vi "Main.vi"(8 "error in (no error)":errorcluster, 11 "RSABase in":refnum<class "RSA.lvclass">) -> (0 "error out":errorcluster, 3 "component":refnum<class "RSA.lvclass">)   [LabVIEW 2012, in "RSA.lvclass"]
doc: "Main VI of the component."
uses:
  RSA.lvclass
  <vilib>/Distrio/Murmex/Murmex/command_enum.ctl
  starting shape.ctl
  RSA.lvclass/RSA.ctl
  <vilib>/Distrio/Murmex/InitialiseMessage/InitialiseMessage.lvclass
  <vilib>/Distrio/Murmex/TerminateMessage/TerminateMessage.lvclass
  <vilib>/Distrio/Murmex/ConfigureMessage/ConfigureMessage.lvclass
  <vilib>/Distrio/Murmex/StartMessage/StartMessage.lvclass
  <vilib>/Distrio/Murmex/Murmex/update_cluster.ctl
  <vilib>/Distrio/Murmex/ResetMessage/ResetMessage.lvclass
  <vilib>/Distrio/Murmex/Murmex/Set configure at initialise.vi
  <vilib>/Distrio/Murmex/Murmex/Set log reference.vi
  <vilib>/Distrio/Murmex/Murmex/Set VI reference.vi
  <vilib>/Distrio/Murmex/Murmex/Get ID.vi
  <vilib>/Distrio/Murmex/Murmex/Murmex.lvclass
  <vilib>/Distrio/Murmex/Message/Message.lvclass
panel:
  in  "button::stop":bool
  in  "button::reset":bool
  in  "button::start":bool
  in  "button::quit":bool
  in  "Tab Control":enum32{"Settings", "Indicators", "Debug"}(tab)
  in  "Starting shape":T1=enum."Midrange"
  in  "BC buffer size":i32=12
  in  "Wait time":dbl[unit]=50.0
  in  "stop after":i32=500
  in  "Iterations until BC":i32=5000
  in  "Search Range [%]":dbl(knob)=100.0 min=0.0 max=100.0 step=5.0 scale=0.0..100.0
  in  "Optimisation name":string="bob"
  out "current MF":cluster{"Y":dbl[], "Y":dbl[]}[](graph)
  out "unsuccessfull iterations":i32
  out "successfull iterations":i32
  out "current Merit Factor":dbl
  out "Iterations since last improvement":i32
  out "max Merit Factor":dbl
  out "BC on":bool
  out "MF standard deviation":dbl
  out "best MF":cluster{"Y":dbl[], "Y":dbl[]}[](graph)
  out "BC counter":i32
  out "log":string="\r\n11:11:41.970 05/12/2013: initialise from AOTF to AOTF\r\n11:11:42.586 05/12/2013: inform from AOTF to AOTF\r\n11:11:43.913 05/12/2013: update from AOTF to AOTF\r\n11:11:45.142 05/12/2013: generic (shutter_off) from AOTF to AOTF\r\n11:11:45.270 05/12/2013: generic (shutter_on) from AOTF to AOTF\r\n11:11:45.902 05/12/2013: generic (shutter_off) from AOTF to AOTF\r\n11:11:45.932 05/12/2013: inspect from AOTF to AOTF\r\n11:11:48.013 05/12/2013: configure from AOTF to AOTF\r\n11:11:52.003 05/12/2013: inform from AOTF to AOTF\r\n11:11:58.521 05/12/2013: initialise from AOTF to AOTF\r\n11:11:58.561 05/12/2013: inform from AOTF to AOTF\r\n11:11:58.695 05/12/2013: inform from AOTF to AOTF\r\n11:12:02.089 05/12/2013: update from AOTF to AOTF\r\n11:12:02.308 05/12/2013: inspect from AOTF to AOTF\r\n11:12:02.364 05/12/2013: inform from AOTF to AOTF\r\n11:12:05.062 05/12/2013: generic (shutter_on) from AOTF to AOTF\r\n11:12:06.690 05/12/2013: update from AOTF to AOTF\r\n11:12:06.909 05/12/2013: inspect from AOTF to AOTF\r\n11:12:06.964 05/12/2013: inform from AOTF to AOTF\r\n11:12:07.770 05/12/2013: update from AOTF to AOTF\r\n11:12:07.989 05/12/2013: inspect from AOTF to AOTF\r\n11:12:08.044 05/12/2013: inform from AOTF to AOTF\r\n11:12:08.627 05/12/2013: update from AOTF to AOTF\r\n11:12:08.846 05/12/2013: inspect from AOTF to AOTF\r\n11:12:08.900 05/12/2013: inform from AOTF to AOTF\r\n11:12:09.290 05/12/2013: update from AOTF to AOTF\r\n11:12:09.508 05/12/2013: inspect from AOTF to AOTF\r\n11:12:09.563 05/12/2013: inform from AOTF to AOTF\r\n11:12:10.154 05/12/2013: update from AOTF to AOTF\r\n11:12:10.373 05/12/2013: inspect from AOTF to AOTF\r\n11:12:10.430 05/12/2013: inform from AOTF to AOTF\r\n11:12:20.953 05/12/2013: update from AOTF to AOTF\r\n11:12:21.172 05/12/2013: inspect from AOTF to AOTF\r\n11:12:21.227 05/12/2013: inform from AOTF to AOTF\r\n11:12:22.057 05/12/2013: update from AOTF to AOTF\r\n11:12:22.276 05/12/2013: inspect from AOTF to AOTF\r\n11:12:22.330 05/12/2013: inform from AOTF to AOTF\r\n11:12:22.841 05/12/2013: update from AOTF to AOTF\r\n11:12:23.060 05/12/2013: inspect from AOTF to AOTF\r\n11:12:23.114 05/12/2013: inform from AOTF to AOTF\r\n11:12:23.449 05/12/2013: update from AOTF to AOTF\r\n11:12:23.668 05/12/2013: inspect from AOTF to AOTF\r\n11:12:23.724 05/12/2013: inform from AOTF to AOTF\r\n11:12:24.514 05/12/2013: update from AOTF to AOTF\r\n11:12:24.733 05/12/2013: inspect from AOTF to AOTF\r\n11:12:24.789 05/12/2013: inform from AOTF to AOTF\r\n11:12:25.098 05/12/2013: update from AOTF to AOTF\r\n11:12:25.317 05/12/2013: inspect from AOTF to AOTF\r\n11:12:25.371 05/12/2013: inform from AOTF to AOTF\r\n11:12:26.482 05/12/2013: update from AOTF to AOTF\r\n11:12:26.701 05/12/2013: inspect from AOTF to AOTF\r\n11:12:26.755 05/12/2013: inform from AOTF to AOTF\r\n11:12:27.154 05/12/2013: update from AOTF to AOTF\r\n11:12:27.373 05/12/2013: inspect from AOTF to AOTF\r\n11:12:27.428 05/12/2013: inform from AOTF to AOTF\r\n11:12:27.666 05/12/2013: update from AOTF to AOTF\r\n11:12:27.885 05/12/2013: inspect from AOTF to AOTF\r\n11:12:27.944 05/12/2013: inform from AOTF to AOTF\r\n11:12:33.380 05/12/2013: update from AOTF to AOTF\r\n11:12:33.484 05/12/2013: update from AOTF to AOTF\r\n11:12:33.603 05/12/2013: inspect from AOTF to AOTF\r\n11:12:33.611 05/12/2013: update from AOTF to AOTF\r\n11:12:33.684 05/12/2013: update from AOTF to AOTF\r\n11:12:33.740 05/12/2013: update from AOTF to AOTF\r\n11:12:33.827 05/12/2013: inspect from AOTF to AOTF\r\n11:12:33.835 05/12/2013: update from AOTF to AOTF\r\n11:12:33.897 05/12/2013: inform from AOTF to AOTF\r\n11:12:33.903 05/12/2013: update from AOTF to AOTF\r\n11:12:33.940 05/12/2013: update from AOTF to AOTF\r\n11:12:34.085 05/12/2013: update from AOTF to AOTF\r\n11:12:34.119 05/12/2013: inspect from AOTF to AOTF\r\n11:12:34.292 05/12/2013: update from AOTF to AOTF\r\n11:12:34.336 05/12/2013: inspect from AOTF to AOTF\r\n11:12:34.553 05/12/2013: inspect from AOTF to AOTF\r\n11:12:34.608 05/12/2013: inform from AOTF to AOTF\r\n11:12:34.739 05/12/2013: update from AOTF to AOTF\r\n11:12:34.771 05/12/2013: update from AOTF to AOTF\r\n11:12:34.826 05/12/2013: inspect from AOTF to AOTF\r\n11:12:34.834 05/12/2013: update from AOTF to AOTF\r\n11:12:34.867 05/12/2013: update from AOTF to AOTF\r\n11:12:34.931 05/12/2013: update from AOTF to AOTF\r\n11:12:34.979 05/12/2013: update from AOTF to AOTF\r\n11:12:35.003 05/12/2013: update from AOTF to AOTF\r\n11:12:35.027 05/12/2013: update from AOTF to AOTF\r\n11:12:35.041 05/12/2013: update from AOTF to AOTF\r\n11:12:35.051 05/12/2013: inspect from AOTF to AOTF\r\n11:12:35.066 05/12/2013: update from AOTF to AOTF\r\n11:12:35.116 05/12/2013: update from AOTF to AOTF\r\n11:12:35.171 05/12/2013: update from AOTF to AOTF\r\n11:12:35.211 05/12/2013: update from AOTF to AOTF\r\n11:12:35.273 05/12/2013: inspect from AOTF to AOTF\r\n11:12:35.287 05/12/2013: update from AOTF to AOTF\r\n11:12:35.475 05/12/2013: update from AOTF to AOTF\r\n11:12:35.495 05/12/2013: inspect from AOTF to AOTF\r\n11:12:35.549 05/12/2013: inform from AOTF to AOTF\r\n11:12:35.764 05/12/2013: inspect from AOTF to AOTF\r\n11:12:35.819 05/12/2013: inform from AOTF to AOTF\r\n11:12:35.861 05/12/2013: update from AOTF to AOTF\r\n11:12:35.877 05/12/2013: inform from AOTF to AOTF\r\n11:12:35.947 05/12/2013: update from AOTF to AOTF\r\n11:12:36.067 05/12/2013: update from AOTF to AOTF\r\n11:12:36.100 05/12/2013: inspect from AOTF to AOTF\r\n11:12:36.235 05/12/2013: update from AOTF to AOTF\r\n11:12:36.317 05/12/2013: inspect from AOTF to AOTF\r\n11:12:36.371 05/12/2013: inform from AOTF to AOTF\r\n11:12:36.587 05/12/2013: inspect from AOTF to AOTF\r\n11:12:36.771 05/12/2013: update from AOTF to AOTF\r\n11:12:36.804 05/12/2013: inspect from AOTF to AOTF\r\n11:12:37.020 05/12/2013: inspect from AOTF to AOTF\r\n11:12:37.238 05/12/2013: inspect from AOTF to AOTF\r\n11:12:37.456 05/12/2013: inspect from AOTF to AOTF\r\n11:12:37.673 05/12/2013: inspect from AOTF to AOTF\r\n11:12:37.891 05/12/2013: inspect from AOTF to AOTF\r\n11:12:37.946 05/12/2013: inform from AOTF to AOTF\r\n11:12:38.161 05/12/2013: inspect from AOTF to AOTF\r\n11:12:38.379 05/12/2013: inspect from AOTF to AOTF\r\n11:12:38.597 05/12/2013: inspect from AOTF to AOTF\r\n11:12:38.815 05/12/2013: inspect from AOTF to AOTF\r\n11:12:38.871 05/12/2013: inform from AOTF to AOTF\r\n11:12:39.086 05/12/2013: inspect from AOTF to AOTF\r\n11:12:39.303 05/12/2013: inspect from AOTF to AOTF\r\n11:12:39.363 05/12/2013: inform from AOTF to AOTF\r\n11:12:39.417 05/12/2013: inform from AOTF to AOTF\r\n11:12:39.633 05/12/2013: inspect from AOTF to AOTF\r\n11:12:39.852 05/12/2013: inspect from AOTF to AOTF\r\n11:12:40.069 05/12/2013: inspect from AOTF to AOTF\r\n11:12:40.124 05/12/2013: inform from AOTF to AOTF\r\n11:12:40.339 05/12/2013: inspect from AOTF to AOTF\r\n11:12:40.395 05/12/2013: inform from AOTF to AOTF\r\n11:12:40.448 05/12/2013: inform from AOTF to AOTF\r\n11:12:40.663 05/12/2013: inspect from AOTF to AOTF\r\n11:12:40.718 05/12/2013: inform from AOTF to AOTF\r\n11:12:40.770 05/12/2013: inform from AOTF to AOTF\r\n11:12:40.824 05/12/2013: inform from AOTF to AOTF\r\n11:12:40.877 05/12/2013: inform from AOTF to AOTF\r\n11:12:40.930 05/12/2013: inform from AOTF to AOTF\r\n11:12:40.982 05/12/2013: inform from AOTF to AOTF\r\n11:12:41.034 05/12/2013: inform from AOTF to AOTF\r\n11:12:41.092 05/12/2013: inform from AOTF to AOTF\r\n11:12:41.144 05/12/2013: inform from AOTF to AOTF\r\n11:12:41.196 05/12/2013: inform from AOTF to AOTF\r\n11:12:41.249 05/12/2013: inform from AOTF to AOTF\r\n11:12:41.307 05/12/2013: inform from AOTF to AOTF\r\n11:12:41.366 05/12/2013: inform from AOTF to AOTF\r\n11:12:41.424 05/12/2013: inform from AOTF to AOTF\r\n11:12:41.478 05/12/2013: inform from AOTF to AOTF\r\n11:12:41.533 05/12/2013: inform from AOTF to AOTF\r\n11:12:41.589 05/12/2013: inform from AOTF to AOTF\r\n11:12:42.246 05/12/2013: terminate from AOTF to AOTF"
  in  "ID":string="RSA"
  in  "command":T2
  in  "Generic command":string
  in  "button::configure":bool
  in  "button::send":bool
  out "terminate?":bool=TRUE
  # "RSA settings"
  # "Save settings"
  # "Bleaching compensation"
  # "Iterations"
  # "Merit Factor"
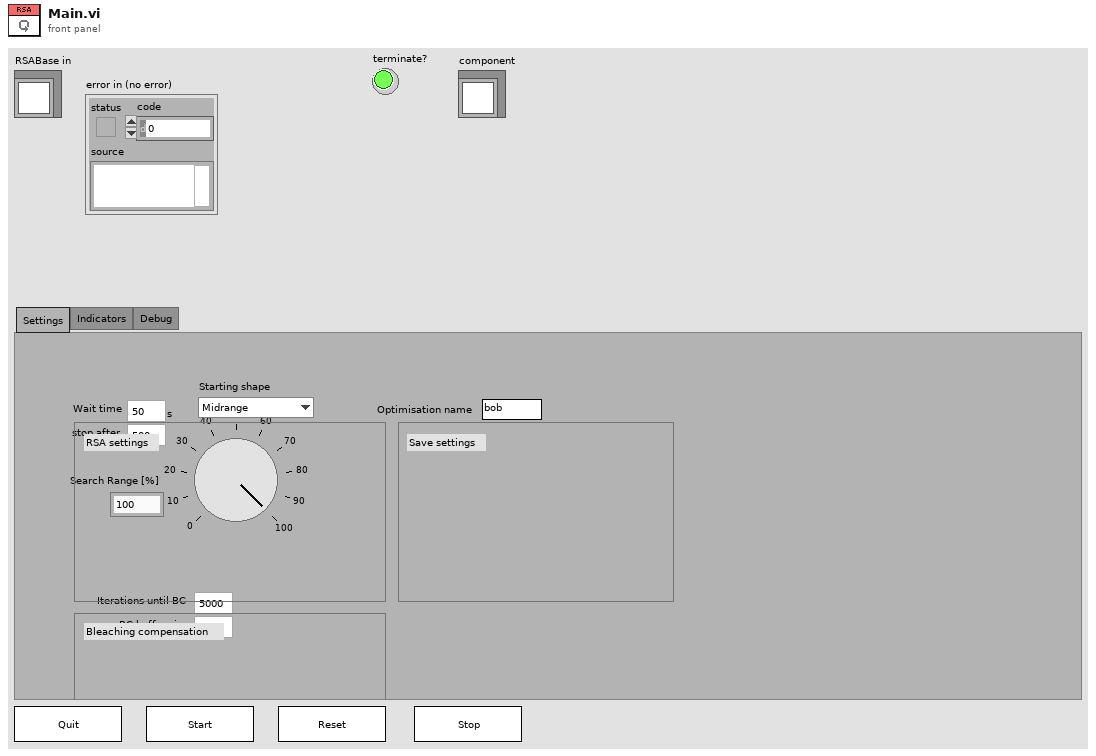
[diagram p1: front panel]
types:
  T1 = typedef "RSA.lvclass/starting shape.ctl" = enum16{"Load shape", "Midrange"}
  T2 = typedef "Murmex.lvlib/Murmex.lvclass/command_enum.ctl" = enum16{"null", "initialise", "reset", "terminate", "acknowledge", "update", "inspect", "inform", "proceed", "start", "stop", "fetch", "configure", "generic"}
  T3 = typedef "Murmex.lvlib/Murmex.lvclass/update_cluster.ctl" = cluster{"target ID":string, "key chains":string[], "values":variant[]}
  T4 = enum8{"Enabled", "Disabled", "Disabled and Grayed Out"}
  T5 = typedef "Murmex.lvclass/command_enum.ctl" = enum16{"null", "initialise", "reset", "terminate", "acknowledge", "update", "inspect", "inform", "proceed", "start", "stop", "fetch", "configure", "generic"}
  T6 = typedef "Murmex.lvclass/Event type enumerations.ctl" = enum16{"before", "after"}
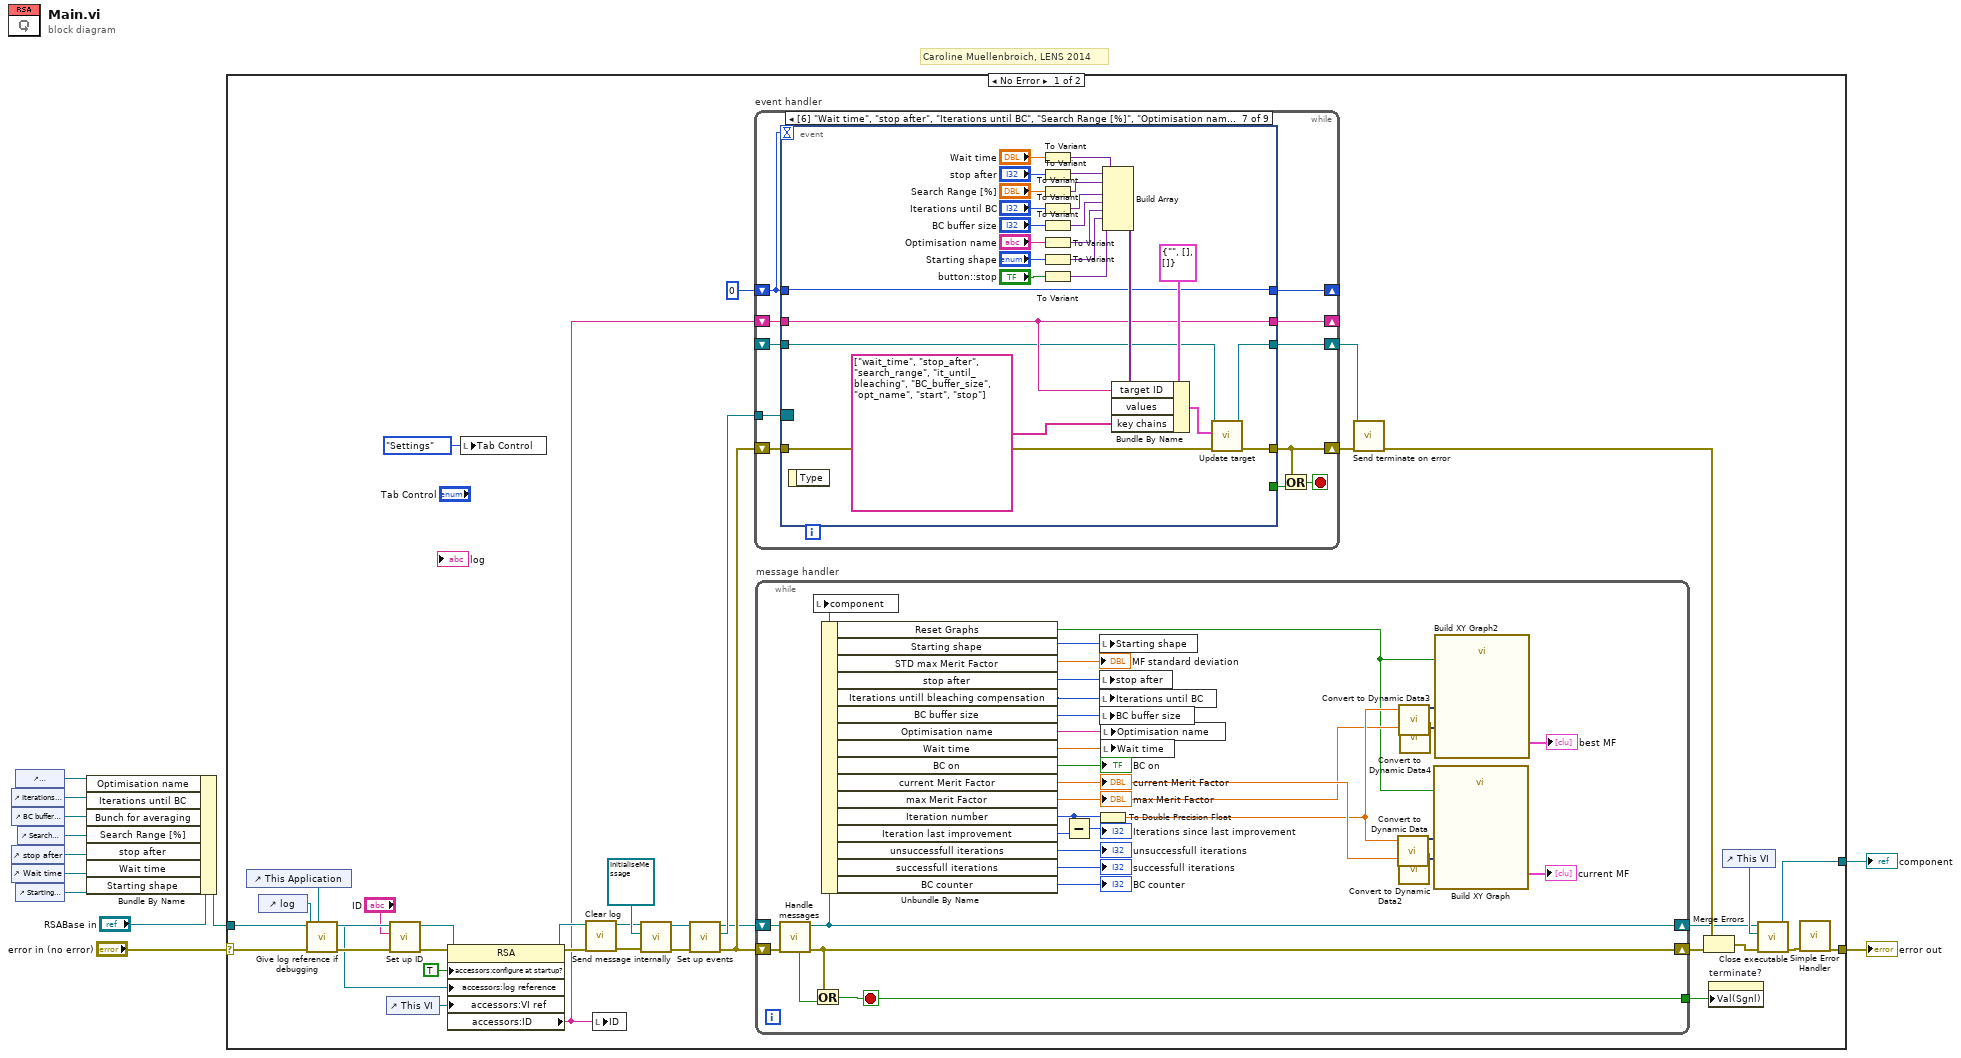
[diagram p0: block diagram]
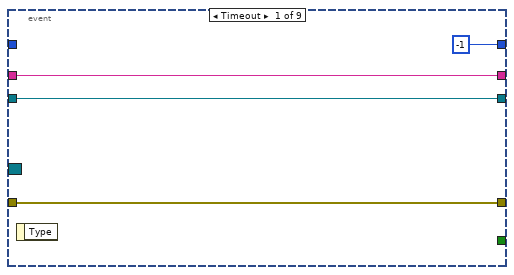
[diagram p2: hidden frame]
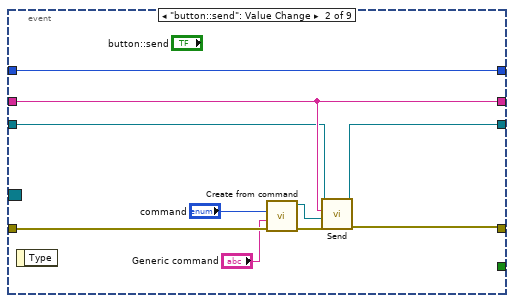
[diagram p3: hidden frame]
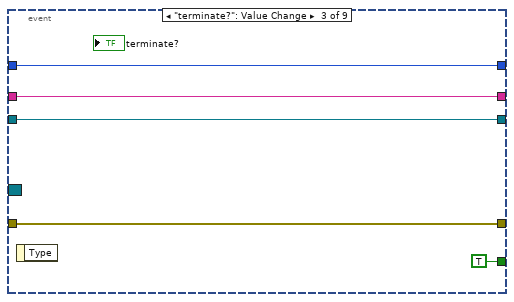
[diagram p4: hidden frame]
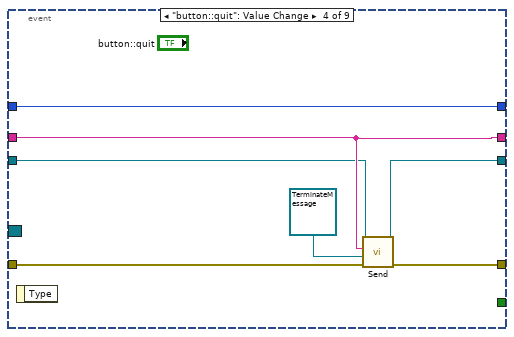
[diagram p5: hidden frame]
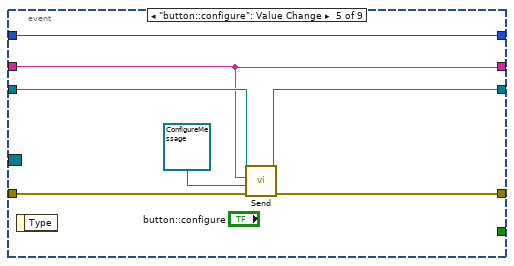
[diagram p6: hidden frame]
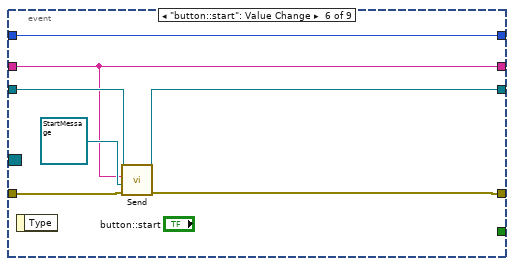
[diagram p7: hidden frame]
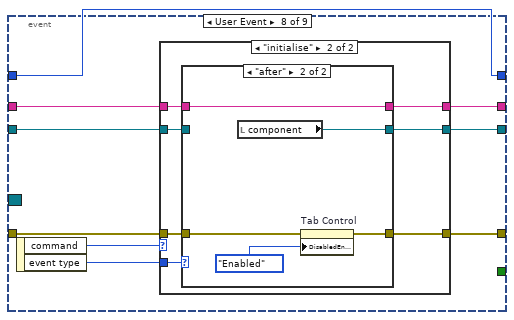
[diagram p8: hidden frame]
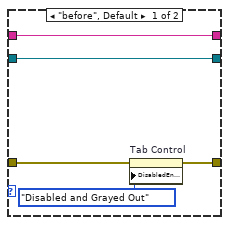
[diagram p10: hidden frame]
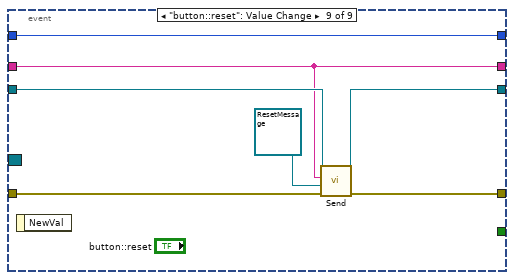
[diagram p11: hidden frame]
diagram:
  # "Caroline Muellenbroich, LENS 2014"
  n1 = control-ref of="Iterations until BC"() -> (w3:refnum<vi>)
  n2 = control-ref of="BC buffer size"() -> (w4:refnum<vi>)
  n3 = control-ref of="stop after"() -> (w6:refnum<vi>)
  n4 = control-ref of="Wait time"() -> (w1:refnum<vi>)
  n5 = control-ref of="Optimisation name"() -> (w2:refnum<vi>)
  n6 = control-ref of="Starting shape"() -> (w7:refnum<vi>)
  n7 = control-ref of="Search Range [%]"() -> (w5:refnum<vi>)
  n8 = Bundle By Name(cluster="RSABase in", "Optimisation name"=w2, "Iterations until BC"=w3, "Bunch for averaging"=w4, "Search Range [%]"=w5, "stop after"=w6, "Wait time"=w1, "Starting shape"=w7) -> (w8:refnum<class "RSA.lvclass">)
  n9 = case shown="No Error" "error in (no error)" {
    selector: "error in (no error)" -> [w19 w192]
    tunnel: w8 -> [w43 w191]
    tunnel: [w25 w191] -> w11
    tunnel: [w23 w192] -> w10
    frame No Error {
      n10 = control-ref of="This Application"() -> (w15:refnum<vi>)
      n11 = control-ref of="log"() -> (w17:refnum<vi>)
      n12 = call "Give log reference if debugging.vi"("application ref"=w15, "error in (no error)"=w19, "log reference in"=w17) -> ("error out"=w18:errorcluster, "log reference out"=w16:refnum<vi>)  [unwired: 6 in, 1 out]
      n13 = control-ref of="This VI"() -> (w47:refnum<vi>)
      n14 = call <vilib>:"Set up ID.vi"("error in (no error)"=w18, "component ID"="ID", "MurmexBase in"=w43) -> ("error out"=w44:errorcluster, "MurmexBase out"=w45:refnum<class "RSA.lvclass">)  [unwired: 6 in, 1 out]
      n15 = property class="RSA"(reference=w45, error in=w44, "accessors:configure at startup?"=TRUE ("configure at startup?"), "accessors:log reference"=w16, "accessors:VI ref"=w47) -> (reference out=w36:refnum<class "RSA.lvclass">, error out=w37:errorcluster, "accessors:ID"=w13:string)
      n16 = local write "Tab Control"(enum32{"Settings", "Indicators", "Debug"}."Settings" ("Tab Control")) -> ()
      n17 = call <vilib>:"Clear log.vi"("error in (no error)"=w37, "MurmexBase in"=w36) -> ("error out"=w38:errorcluster, "MurmexBase out"=w39:refnum<class "RSA.lvclass">)  [unwired: 8 in]
      n18 = local write "ID"(w13) -> ()
      n19 = call <vilib>:"Send message internally.vi"("error in (no error)"=w38, "Message"=refnum<class "InitialiseMessage.lvclass"> refnum ("Murmex.lvlib:InitialiseMessage"), "Murmex in"=w39) -> ("error out"=w40:errorcluster, "Murmex out"=w41:refnum<class "RSA.lvclass">)  [unwired: 7 in]
      n20 = call <vilib>:"Set up events.vi"("error in (no error)"=w40, "MurmexBase in"=w41) -> ("error out"=w34:errorcluster, "Event Registration Refnum"=w35:refnum<event-registration>, "MurmexBase out"=w33:refnum<class "RSA.lvclass">)  [unwired: 7 in]
      n21 = while "event handler" {
        shift-right: [w84] -> _
        shift-left: w13 -> [w87]
        shift-right: [w83] -> w31
        shift-left: w34 -> [w88]
        shift-right: [w85] -> _
        shift-left: 0 -> [w86]
        shift-right: [w80] -> w22
        shift-left: _ -> [w79]
        tunnel: w35 -> [w81]
        stop <- w82 stop-if-true
        n22 = event shown="[6] \"Wait time\", \"stop after\", \"Iterations until BC\", \"Search Range [%]\", \"Optimisation name\", \"BC buffer size\", \"Starting shape\", \"button::stop\": Value Change" {
          selector: w81 -> [_ _ _ _ _ _ _ _ _]
          dyn-events: _ -> [_ _ _ _ _ _ _ _ _]
          timeout: w86 -> [_ _ _ _ _ _ _ _ _]
          tunnel: w88 -> [w90 w100 w103 w113 w120 w128 w154 w158 w190]
          tunnel: w87 -> [w91 w96 w105 w111 w116 w123 w143 w161 w185]
          tunnel: w86 -> [_ w93 w106 w108 w115 w122 w142 w159 w184]
          tunnel: [-1 w93 w106 w108 w115 w122 w142 w159 w184] -> w85
          tunnel: [w91 w96 w105 w111 w116 w123 w143 w160 w185] -> w84
          tunnel: [w90 w99 w103 w112 w119 w127 w153 w157 w189] -> w83
          tunnel: [w89 w94 w104 w109 w117 w124 w147 w156 w186] -> w80
          tunnel: w79 -> [w89 w95 w104 w110 w118 w125 w135 w155 w187]
          tunnel: [_ _ TRUE _ _ _ _ _ _] -> w78
          event Timeout {
            n23 = event-data() -> ()  [unwired: 1 in, 1 out]
          }
          event "button::send": Value Change {
            n24 = event-data() -> ()  [unwired: 1 in, 1 out]
            n25 = call <vilib>:"Create from command.vi"("error in (no error)"=w100, "generic command"="Generic command", "command"="command") -> ("error out"=w101:errorcluster, "Message out"=w102:refnum<class "Message.lvclass">)  [unwired: 7 in]
            n26 = call <vilib>:"Send.vi"("error in (no error)"=w101, "Message"=w102, "recipient"=w96, "Murmex in"=w95) -> ("error out"=w99:errorcluster, "Murmex out"=w94:refnum<class "RSA.lvclass">)  [unwired: 6 in]
          }
          event "terminate?": Value Change {
            n27 = event-data() -> ()  [unwired: 1 in, 1 out]
          }
          event "button::quit": Value Change {
            n28 = event-data() -> ()  [unwired: 1 in, 1 out]
            n29 = call <vilib>:"Send.vi"("error in (no error)"=w113, "Message"=refnum<class "TerminateMessage.lvclass"> refnum ("Murmex.lvlib:TerminateMessage"), "recipient"=w111, "Murmex in"=w110) -> ("error out"=w112:errorcluster, "Murmex out"=w109:refnum<class "RSA.lvclass">)  [unwired: 6 in]
          }
          event "button::configure": Value Change {
            n30 = event-data() -> ()  [unwired: 1 in, 1 out]
            n31 = call <vilib>:"Send.vi"("error in (no error)"=w120, "Message"=refnum<class "ConfigureMessage.lvclass"> refnum ("Murmex.lvlib:ConfigureMessage"), "recipient"=w116, "Murmex in"=w118) -> ("error out"=w119:errorcluster, "Murmex out"=w117:refnum<class "RSA.lvclass">)  [unwired: 6 in]
          }
          event "button::start": Value Change {
            n32 = event-data() -> ()  [unwired: 1 in, 1 out]
            n33 = call <vilib>:"Send.vi"("error in (no error)"=w128, "Message"=refnum<class "StartMessage.lvclass"> refnum ("Message in"), "recipient"=w123, "Murmex in"=w125) -> ("error out"=w127:errorcluster, "Murmex out"=w124:refnum<class "RSA.lvclass">)  [unwired: 6 in]
          }
          event "Wait time", "stop after", "Iterations until BC", "Search Range [%]", "Optimisation name", "BC buffer size", "button::stop": Value Change {
            n34 = event-data() -> ()  [unwired: 1 in, 1 out]
            n35 = To Variant(anything="Wait time") -> (Variant=w149:variant)
            n36 = To Variant(anything="stop after") -> (Variant=w152:variant)
            n37 = To Variant(anything="Search Range [%]") -> (Variant=w151:variant)
            n38 = To Variant(anything="Iterations until BC") -> (Variant=w150:variant)
            n39 = To Variant(anything="BC buffer size") -> (Variant=w137:variant)
            n40 = To Variant(anything="Optimisation name") -> (Variant=w138:variant)
            n41 = To Variant(anything="Starting shape") -> (Variant=w133:variant)
            n42 = To Variant(anything="button::stop") -> (Variant=w129:variant)
            n43 = Build Array(w149, w152, w151, w150, w137, w138, w133, w129) -> (w146:variant[])
            n44 = Bundle By Name(cluster=T3 {"target ID"="", "key chains"=[], "values"=[]} ("update cluster"), "target ID"=w143, "values"=w146, "key chains"=string[] ["wait_time", "stop_after", "search_range", "it_until_bleaching", "BC_buffer_size", "opt_name", "start", "stop"]) -> (w148:T3)
            n45 = call <vilib>:"Update target.vi"("error in (no error)"=w154, "update cluster"=w148, "MurmexBase in"=w135) -> ("error out"=w153:errorcluster, "MurmexBase out"=w147:refnum<class "RSA.lvclass">)  [unwired: 7 in]
          }
          event User Event {
            n46 = event-data() -> ("command"=w163:T5, "event type"=w162:T6)  [unwired: 1 in]
            n47 = case shown="\"initialise\"" w163 {
              tunnel: w162 -> [_ w173]
              tunnel: w161 -> [w166 w172]
              tunnel: [w166 w171] -> w160
              tunnel: w158 -> [w165 w170]
              tunnel: [w165 w169] -> w157
              tunnel: [w164 w168] -> w156
              tunnel: w155 -> [w164 w167]
              frame "null", Default {
              }
              frame "initialise" {
                n48 = case shown="\"after\"" w173 {
                  tunnel: w172 -> [w178 w183]
                  tunnel: [w178 w183] -> w171
                  tunnel: w170 -> [w175 w181]
                  tunnel: [w174 w180] -> w169
                  tunnel: [w177 w182] -> w168
                  tunnel: w167 -> [w177 _]
                  frame "before", Default {
                    n49 = property on="Tab Control" class="TabCtl (strict)"(error in=w175, "DisabledEnum"=T4."Disabled and Grayed Out" ("Disabled")) -> (error out=w174:errorcluster)  [unwired: 1 in, 1 out]
                  }
                  frame "after" {
                    n50 = local read "component"() -> (w182:refnum<class "RSA.lvclass">)
                    n51 = property on="Tab Control" class="TabCtl (strict)"(error in=w181, "DisabledEnum"=T4."Enabled" ("Disabled")) -> (error out=w180:errorcluster)  [unwired: 1 in, 1 out]
                  }
                }
              }
            }
          }
          event "button::reset": Value Change {
            n52 = event-data() -> ()  [unwired: 1 in, 1 out]
            n53 = call <vilib>:"Send.vi"("error in (no error)"=w190, "Message"=refnum<class "ResetMessage.lvclass"> refnum ("Distrio Murmex 1.0:ResetMessage"), "recipient"=w185, "Murmex in"=w187) -> ("error out"=w189:errorcluster, "Murmex out"=w186:refnum<class "RSA.lvclass">)  [unwired: 6 in]
          }
        }
        n54 = Or(x=w83, y=w78) -> (x .or. y?=w82:bool)
      }
      n55 = while "message handler" {
        shift-right: [w74] -> w30
        shift-left: w34 -> [w76]
        shift-right: [w50] -> w26
        shift-left: w33 -> [w75]
        tunnel: [w73] -> w20
        stop <- w73 stop-if-true
        n56 = call <vilib>:"Handle messages.vi"("error in (no error)"=w76, "Murmex in"=w75) -> ("error out"=w74:errorcluster, "Murmex out"=w50:refnum<class "RSA.lvclass">, "terminated?"=w77:bool)  [unwired: 7 in]
        n57 = Or(x=w74, y=w77) -> (x .or. y?=w73:bool)
        n58 = local write "component"(w50) -> ()
        n59 = Unbundle By Name(w50) -> ("Reset Graphs"=w48:bool, "Starting shape"=w49:T1, "STD max Merit Factor"=→"MF standard deviation":dbl, "stop after"=w59:i32, "Iterations untill bleaching compensation"=w58:i32, "BC buffer size"=w60:i32, "Optimisation name"=w61:string, "Wait time"=w62:dbl[unit], "BC on"=→"BC on":bool, "current Merit Factor"=w63:dbl, "max Merit Factor"=w52:dbl, "Iteration number"=w66:i32, "Iteration last improvement"=w72:i32, "unsuccessfull iterations"=→"unsuccessfull iterations":i32, "successfull iterations"=→"successfull iterations":i32, "BC counter"=→"BC counter":i32)
        "current Merit Factor" <- w63
        "max Merit Factor" <- w52
        n60 = Subtract(x=w66, y=w72) -> (x-y=→"Iterations since last improvement":i32)
        n61 = To Double Precision Float(number=w66) -> (double precision float=w54:dbl)
        n62 = local write "Starting shape"(w49) -> ()
        n63 = local write "stop after"(w59) -> ()
        n64 = local write "Iterations until BC"(w58) -> ()
        n65 = local write "BC buffer size"(w60) -> ()
        n66 = local write "Optimisation name"(w61) -> ()
        n67 = local write "Wait time"(w62) -> ()
        n68 = call "Convert to Dynamic Data"("Double"=w54) -> ("Dynamic Data Type"=w65:dynamicdata)  [unwired: 3 in]
        n69 = call "Convert to Dynamic Data3"("Double"=w54) -> ("Dynamic Data Type"=w56:dynamicdata)  [unwired: 3 in]
        n70 = call "Convert to Dynamic Data2"("Double"=w63) -> ("Dynamic Data Type"=w64:dynamicdata)  [unwired: 3 in]
        n71 = call "Convert to Dynamic Data4"("Double"=w52) -> ("Dynamic Data Type"=w57:dynamicdata)  [unwired: 3 in]
        n72 = call "Build XY Graph"("Reset"=w48, "Y Input"=w64, "X Input"=w65) -> ("XY Graph"=→"current MF":cluster{"Y":dbl[], "Y":dbl[]}[])  [unwired: 2 in, 6 out]
        n73 = call "Build XY Graph2"("Reset"=w48, "Y Input"=w57, "X Input"=w56) -> ("XY Graph"=→"best MF":cluster{"Y":dbl[], "Y":dbl[]}[])  [unwired: 2 in, 6 out]
      }
      n74 = call <vilib>:"Send terminate on error.vi"("error in (no error)"=w31, "Murmex in"=w22) -> ("error out"=w29:errorcluster)  [unwired: 8 in, 1 out]
      n75 = Merge Errors(w29, w30) -> (w28:errorcluster)
      n76 = property on="terminate?" class="Bool (strict)"("Val(Sgnl)"=w20) -> ()  [unwired: 2 in, 2 out]
      n77 = control-ref of="This VI"() -> (w27:refnum<vi>)
      n78 = call <vilib>:"Close executable.vi"("error in (no error)"=w28, "main VI ref (optional)"=w27, "MurmexBase in"=w26) -> ("error out"=w24:errorcluster, "MurmexBase out"=w25:refnum<class "RSA.lvclass">)  [unwired: 7 in]
      n79 = call <vilib>:"Simple Error Handler.vi"("error in (no error)"=w24) -> ("error out"=w23:errorcluster)  [unwired: 4 in, 4 out]
    }
    frame Error {
    }
  }
  "error out" <- w10
  "component" <- w11
